vi "Configure Waveform (Constant Dwell).vi"(0 "VISA resource name":refnum<visa-resource-name>, 1 "Dwell Time (0.001 s)":dbl=0.001 format="%^.3e", 5 "Channel Name (1)":string="1", 7 "Constant Dwell Level":dbl[](array[numeric]) format="%^.3e", 9 "Waveform Type (1: Voltage)":i32(ring)=1 items=["Voltage"=1, "Current"=0], 11 "error in (no error)":errorcluster {"code" format="%.0x"}) -> (4 "VISA resource name out":refnum<visa-resource-name>, 15 "error out":errorcluster {"code" format="%.0x"})   [LabVIEW 2014, in "Agilent N6700 Series.lvlib"]
doc: "Configures the constant dwell waveform.\n\n<b>Note:</b>\nThis VI only applies to the N6705B and N6705C DC Power Analyzer."
uses:
  Agilent N6700 Series.lvlib
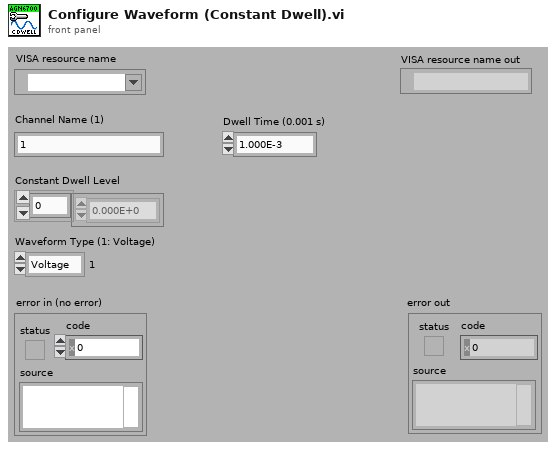
[diagram p1: front panel]
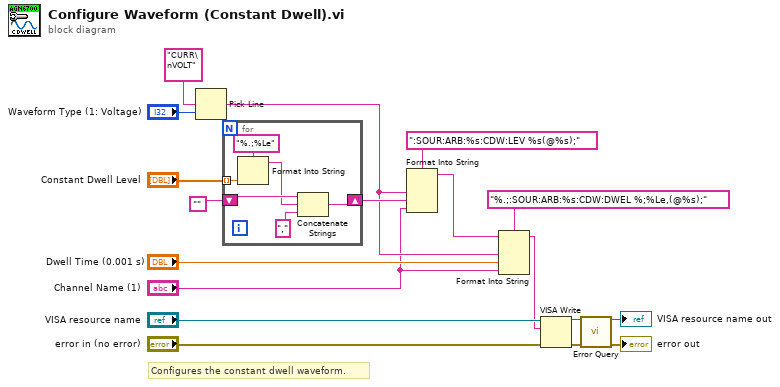
[diagram p0: block diagram]
diagram:
  # "Configures the constant dwell waveform."
  n1 = Pick Line(multi-line string="CURR\nVOLT", line index="Waveform Type (1: Voltage)") -> (output string=w3:string)  [unwired: 1 in]
  n2 = for {
    tunnel: "Constant Dwell Level" -> [w20] mode=indexing
    shift-right: [w24] -> w9
    shift-left: "" ("Empty String Constant") -> [w23]
    n3 = Format Into String(format string="%.;%Le", w20) -> (resulting string=w19:string)  [unwired: 2 in, 1 out]
    n4 = Concatenate Strings(w23, w19, ",") -> (w24:string)
  }
  n5 = Format Into String(format string=":SOUR:ARB:%s:CDW:LEV %s(@%s);", w3, w9, "Channel Name (1)") -> (resulting string=w4:string)  [unwired: 2 in, 1 out]
  n6 = Format Into String(format string="%.;:SOUR:ARB:%s:CDW:DWEL %;%Le,(@%s);", initial string=w4, w3, "Dwell Time (0.001 s)", "Channel Name (1)") -> (resulting string=w1:string)  [unwired: 1 in, 1 out]
  n7 = VISA Write(VISA resource name="VISA resource name", write buffer=w1, error in (no error)="error in (no error)") -> (VISA resource name out=w11:refnum<visa-resource-name>, error out=w10:errorcluster)  [unwired: 1 out]
  n8 = call "Error Query.vi"("VISA resource name"=w11, "error in (no error)"=w10) -> ("VISA resource name out"=→"VISA resource name out":refnum<visa-resource-name>, "error out"=→"error out":errorcluster)  [unwired: 10 in, 2 out]
